vi "PH_Stepmotor_BaseClass.Axis DIM update Information Service.vi"(3 "error in (no error)":errorcluster, 4 "Axis Information":T2, 5 "Axis DIM IDs":T1) -> (0 "error out":errorcluster)   [LabVIEW 2014, in "PH_Stepmotor_BaseClass.lvlib"]
uses:
  PH_Stepmotor_BaseClass.lvlib
  PH_Stepmotor_BaseClass.Axis Information.ctl
  PH_Stepmotor_BaseClass.Axis Activity.ctl
  PH_Stepmotor_BaseClass.Axis DIM Service IDs.ctl
  lib.lib/DimLVEvent/LVDimInterface/LVDimInterface.lvlib
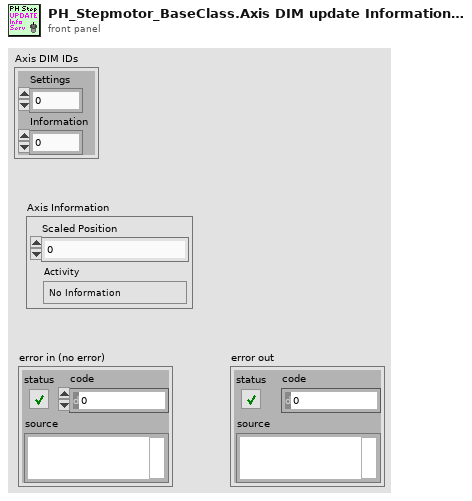
[diagram p1: front panel]
types:
  T1 = typedef "PH_Stepmotor_BaseClass.lvlib/PH_Stepmotor_BaseClass.Axis DIM Service IDs.ctl" = cluster{"Settings":i32, "Information":i32}
  T2 = typedef "PH_Stepmotor_BaseClass.lvlib/PH_Stepmotor_BaseClass.Axis Information.ctl" = cluster{"Scaled Position":dbl, "Activity":T3}
  T3 = typedef "PH_Stepmotor_BaseClass.lvlib/PH_Stepmotor_BaseClass.Axis Activity.ctl" = enum16{"No Information", "stopped", "running", "Failure", "Alarm", "stopped at backward ES", "stopped at foreward ES"}
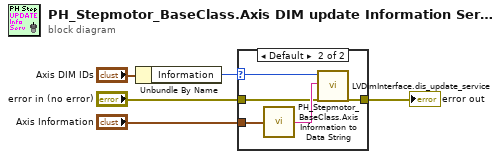
[diagram p0: block diagram]
diagram:
  n1 = Unbundle By Name("Axis DIM IDs") -> ("Information"=w1:i32)
  n2 = case shown="Default" w1 {
    selector: w1 -> [_ w8]
    tunnel: [w6 w11] -> w2
    tunnel: "Axis Information" -> [_ w10]
    tunnel: "error in (no error)" -> [w6 w7]
    frame -1 {
    }
    frame Default {
      n3 = call "PH_Stepmotor_BaseClass.Axis Information to Data String.vi"("Axis Information"=w10) -> ("Data String"=w9:string)
      n4 = call "LVDimInterface.dis_update_service.vi"("my_serviceID"=w8, "data"=w9, "error in (no error)"=w7) -> ("error out"=w11:errorcluster)  [unwired: 14 in, 2 out]
    }
  }
  "error out" <- w2
